vi "CronScheduler.vi"(8 "error in (no error)":errorcluster, 9 "chron schedule":T1={"minutes"="*", "hours"="*", "day of month"="*", "month"="*", "day of week"="*", "year"="*"}, 10 "timestamp":timestamp, 11 "cron id":string) -> (0 "error out":errorcluster, 3 "event elapsed":bool)   [LabVIEW 2017, in "CronScheduler.lvlib"]
doc: "This VI uses CRON strings to evaluate if a time event has occurred. Supported parsing indicators are:\n\",\" - multiple\n\"/\" - increment\n\"-\" - range\n\"*\" - any\n\nExamples:\nminutes field: 1,4,*/15 \nThis expression will be true on the 1st and 4th minute as well as every 15th minute starting at zero.\n\nValid values:\nminutes -> 0 - 59\nhours -> 0 -23\nday of month -> 1-31\nmonth -> 1 - 12\nday of week -> 0 - 6\nyear -> 1970 - 4099"
uses:
  <vilib>/addons/InsightCM/Utilities/CronScheduler/CronScheduler.lvlib
  <vilib>/addons/InsightCM/Utilities/CronScheduler/controls/CronSchedule.ctl
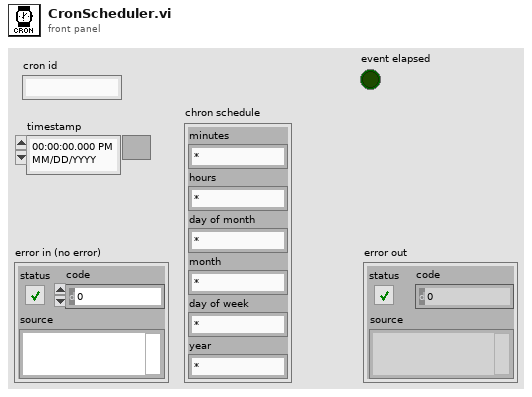
[diagram p1: front panel]
types:
  T1 = typedef "CronScheduler.lvlib/CronSchedule.ctl" = cluster{"minutes":string, "hours":string, "day of month":string, "month":string, "day of week":string, "year":string}
  T2 = typedef "LVDateTimeRec.ctl" = cluster{"fractional second":dbl, "second":i32, "minute":i32, "hour":i32, "day of month":i32, "month":i32, "year":i32, "day of week":i32, "day of year":i32, "DST":i32}
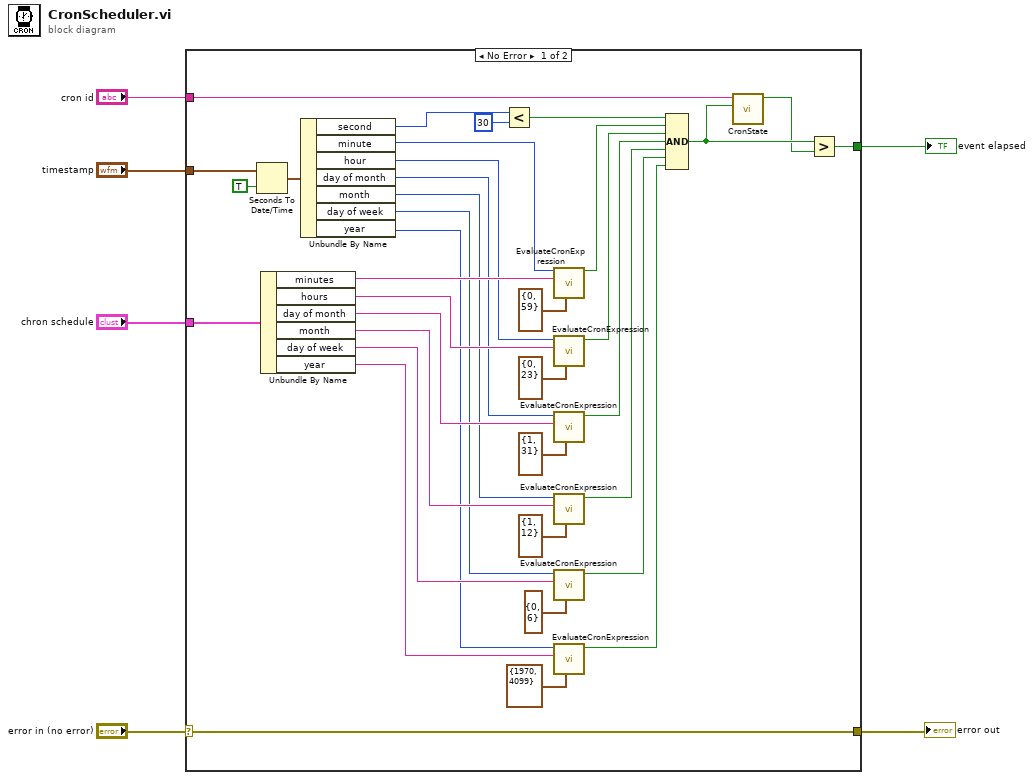
[diagram p0: block diagram]
diagram:
  n1 = case shown="No Error" "error in (no error)" {
    selector: "error in (no error)" -> [w42 w43]
    tunnel: [w42 w43] -> w5
    tunnel: "chron schedule" -> [w40 _]
    tunnel: "timestamp" -> [w11 _]
    tunnel: [w41 _] -> w2
    tunnel: "cron id" -> [w39 _]
    frame No Error {
      n2 = Seconds To Date/Time(time stamp (now)=w11, to UTC (F)=TRUE) -> (date time rec=w38:T2)
      n3 = Unbundle By Name(w40) -> ("minutes"=w36:string, "hours"=w32:string, "day of month"=w28:string, "month"=w25:string, "day of week"=w22:string, "year"=w16:string)
      n4 = Unbundle By Name(w38) -> ("second"=w10:i32, "minute"=w37:i32, "hour"=w29:i32, "day of month"=w21:i32, "month"=w20:i32, "day of week"=w19:i32, "year"=w15:i32)
      n5 = Less?(x=w10, y=30) -> (x < y?=w8:bool)
      n6 = call <vilib>:"EvaluateCronExpression.vi"("valid range"=cluster{"start":u32, "end":u32} {"start"=0, "end"=59}, "expression"=w36, "value"=w37) -> ("output"=w34:bool)  [unwired: 7 in, 1 out]
      n7 = call <vilib>:"EvaluateCronExpression.vi"("valid range"=cluster{"start":u32, "end":u32} {"start"=0, "end"=23}, "expression"=w32, "value"=w29) -> ("output"=w31:bool)  [unwired: 7 in, 1 out]
      n8 = call <vilib>:"EvaluateCronExpression.vi"("valid range"=cluster{"start":u32, "end":u32} {"start"=1, "end"=31}, "expression"=w28, "value"=w21) -> ("output"=w27:bool)  [unwired: 7 in, 1 out]
      n9 = call <vilib>:"EvaluateCronExpression.vi"("valid range"=cluster{"start":u32, "end":u32} {"start"=1, "end"=12}, "expression"=w25, "value"=w20) -> ("output"=w24:bool)  [unwired: 7 in, 1 out]
      n10 = call <vilib>:"EvaluateCronExpression.vi"("valid range"=cluster{"start":u32, "end":u32} {"start"=0, "end"=6}, "expression"=w22, "value"=w19) -> ("output"=w18:bool)  [unwired: 7 in, 1 out]
      n11 = call <vilib>:"EvaluateCronExpression.vi"("valid range"=cluster{"start":u32, "end":u32} {"start"=1970, "end"=4099}, "expression"=w16, "value"=w15) -> ("output"=w14:bool)  [unwired: 7 in, 1 out]
      n12 = Compound Arithmetic op=AND(w8, w34, w31, w27, w24, w18, w14) -> (w13:bool)
      n13 = call <vilib>:"CronState.vi"("new value"=w13, "cron id"=w39) -> ("previous"=w12:bool)  [unwired: 9 in]
      n14 = Greater?(x=w13, y=w12) -> (0:w41:bool)
    }
    frame Error {
    }
  }
  "error out" <- w5
  "event elapsed" <- w2
